vi "updateDisplay.vi"(8 "error in (no error)":errorcluster, 11 "WinX32Settings in":refnum<class "WinX32Settings.lvclass">) -> (0 "error out":errorcluster, 3 "WinX32Settings out":refnum<class "WinX32Settings.lvclass">)   [LabVIEW 2011, in "Tools.lvlib" / "Settings.lvlib" / "WinX32Settings.lvclass"]
uses:
  WinX32Settings.lvclass
  WinX32Settings.lvclass/WinX32Settings.ctl
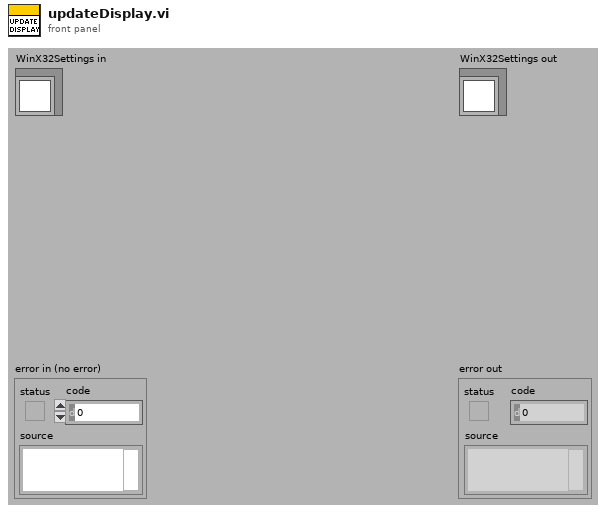
[diagram p1: front panel]
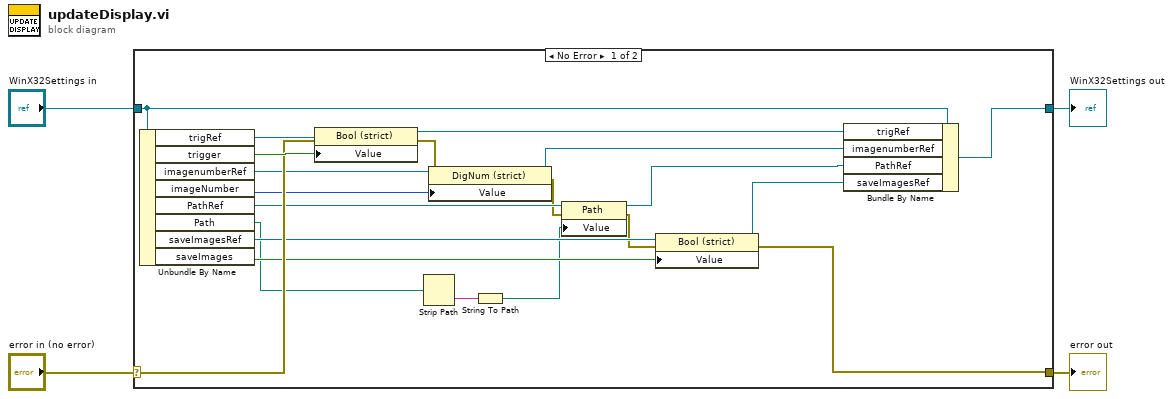
[diagram p0: block diagram]
diagram:
  n1 = case shown="No Error" "error in (no error)" {
    selector: "error in (no error)" -> [w23 w27]
    tunnel: [w10 w27] -> w3
    tunnel: [w8 w26] -> w1
    tunnel: "WinX32Settings in" -> [w9 w26]
    frame No Error {
      n2 = Unbundle By Name(w9) -> ("trigRef"=w25:refnum<vi>, "trigger"=w24:bool, "imagenumberRef"=w22:refnum<vi>, "imageNumber"=w20:i32, "PathRef"=w19:refnum<vi>, "Path"=w6:path, "saveImagesRef"=w17:refnum<vi>, "saveImages"=w15:bool)
      n3 = property class="Bool (strict)"(reference=w25, error in=w23, "Value"=w24) -> (reference out=w14:refnum<vi>, error out=w21:errorcluster)
      n4 = Strip Path(path=w6) -> (name=w7:string)  [unwired: 1 out]
      n5 = property class="DigNum (strict)"(reference=w22, error in=w21, "Value"=w20) -> (reference out=w13:refnum<vi>, error out=w18:errorcluster)
      n6 = String To Path(string=w7) -> (path=w5:path)
      n7 = property class="Path"(reference=w19, error in=w18, "Value"=w5) -> (reference out=w12:refnum<vi>, error out=w16:errorcluster)
      n8 = property class="Bool (strict)"(reference=w17, error in=w16, "Value"=w15) -> (reference out=w11:refnum<vi>, error out=w10:errorcluster)
      n9 = Bundle By Name(cluster=w9, "trigRef"=w14, "imagenumberRef"=w13, "PathRef"=w12, "saveImagesRef"=w11) -> (w8:refnum<class "WinX32Settings.lvclass">)
    }
    frame Error {
    }
  }
  "error out" <- w3
  "WinX32Settings out" <- w1
